vi "fn Read Item SGL.vi"(8 "error in (no error)":errorcluster, 11 "idx":i32) -> (0 "error out":errorcluster, 3 "function return":sgl)   [LabVIEW 2018, in "LV_OPC.lvlib"]
doc: "LVOPC_API float fnReadItemSGL(int idx);"
uses:
  LV_OPC.lvlib
  LVOPC64.dll
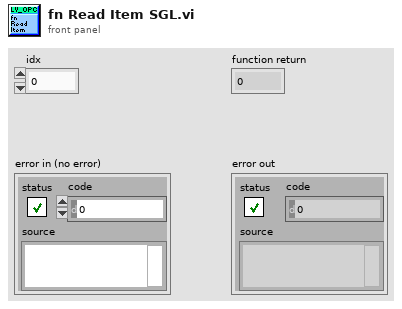
[diagram p1: front panel]
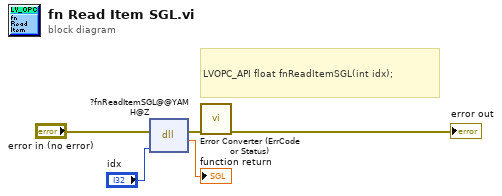
[diagram p0: block diagram]
diagram:
  # "LVOPC_API float fnReadItemSGL(int idx);"
  n1 = dll-call lib="C:/Users/Andrey/Desktop/LV_OPC-Client-x64/LV_OPC_Test/OPC.DLL/LVOPC64.*" fn="?fnReadItemSGL@@YAMH@Z"(error in="error in (no error)", "idx"="idx") -> (error out=w2:errorcluster, "return type"=→"function return":sgl)  [unwired: 3 in, 1 out]
  n2 = call "Error Converter (ErrCode or Status).vi"("error in (no error)"=w2) -> ("error out"=→"error out":errorcluster)  [unwired: 10 in]
